vi "Experiment header-bundle basic image meta data.vi"(11 "AOL_Globals":T1 {"Plane Mode" items=["XY Plane", "XZ Plane", "YZ Plane", "arbitraryplane"]; "Frame Size" items=["100X100"=100, "128X128"=128, "200X200"=200, "256X256"=256, "512X512"=512, "1024x1024"=1024, "2048x2048"=2048]; "Back Apperture (mA)" format="%#.6g"; "Pockels (V)" format="%#.6g"; "PMT 2" format="%#.6g"; "PMT 1" format="%#.6g"; "Angle (degrees)" format="%#.6g"; "POI Dwell time (us)" format="%#.6g"}) -> (3 "Basic image meta-data":T7 {"Frame Size" items=["100X100"=100, "128X128"=128, "200X200"=200, "256X256"=256, "512X512"=512, "1024x1024"=1024, "2048x2048"=2048]})   [LabVIEW 2017]
uses:
  Typedefs/Header subclusters/Header params-Basic image meta data.ctl
  Typedefs/Frame Size.ctl
  Typedefs/Controls/AOL_Globals.ctl
  Typedefs/Imaging Protocols enum.ctl
  Typedefs/AOL modes.ctl
  Typedefs/Plane Mode.ctl
  Typedefs/Functional Mode.ctl
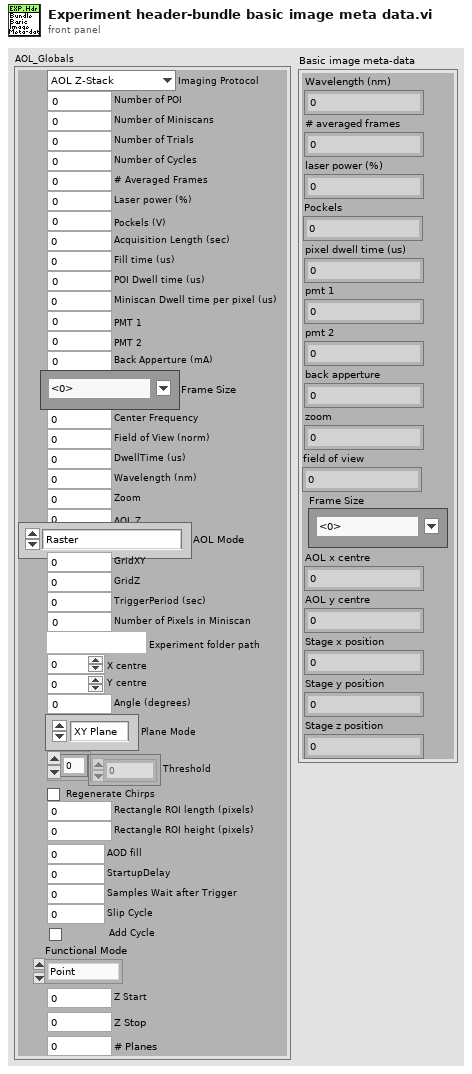
[diagram p1: front panel]
types:
  T1 = typedef "AOL_Globals.ctl" = cluster{"Imaging Protocol":T2, "Number of POI":u16, "Number of Miniscans":u16, "Number of Trials":u16, "Number of Cycles ":u64, "# Averaged Frames":u16, "Laser power (%)":u8, "Pockels (V)":dbl, "Acquisition Length (sec)":dbl, "Fill time (us)":dbl, "POI Dwell time (us)":dbl, "Miniscan Dwell time per pixel (us)":dbl, "PMT 1":dbl, "PMT 2":dbl, "Back Apperture (mA)":dbl, "Frame Size":T3, "Center Frequency":dbl, "Field of View (norm)":dbl, "DwellTime (us)":dbl, "Wavelength (nm)":dbl, "Zoom":dbl, "AOL Z":dbl, "AOL Mode":T4, "GridXY":dbl, "GridZ":dbl, "TriggerPeriod (sec)":dbl, "Number of Pixels in Miniscan":u16, "Experiment folder path":path, "X centre":dbl, "Y centre":dbl, "Angle (degrees)":dbl, "Plane Mode":T5, "Threshold":u16[], "Regenerate Chirps":bool, "Rectangle ROI length (pixels)":u16, "Rectangle ROI height (pixels)":u16, "AOD fill":u16, "StartupDelay":i32, "Samples Wait after Trigger":u16, "Slip Cycle":u32, "Add Cycle":bool, "Functional Mode":T6, "Z Start":dbl, "Z Stop":dbl, "# Planes":i32}
  T2 = typedef "Imaging Protocols enum.ctl" = enum16{"AOL Z-Stack", "Motor Z Stack", "Functional Acquisition", "Single Plane Acquisition", "Volume Acquisition", "Live Imaging", "Live Plane Imaging", "Live Volume Imaging"}
  T3 = typedef "Frame Size.ctl" = u16
  T4 = typedef "AOL modes.ctl" = enum16{"Raster", "Structural", "Pointing", "Mini Scan", "Alignment"}
  T5 = typedef "Plane Mode.ctl" = u16
  T6 = typedef "Functional Mode.ctl" = enum16{"Point", "Line", "Patch", "Plane", "Volume"}
  T7 = typedef "Header params-Basic image meta data.ctl" = cluster{"Wavelength (nm)":dbl, "# averaged frames":dbl, "laser power (%)":dbl, "Pockels":dbl, "pixel dwell time (us)":dbl, "pmt 1":dbl, "pmt 2":dbl, "back apperture":dbl, "zoom":dbl, "field of view":dbl, "Frame Size":T3, "AOL x centre":dbl, "AOL y centre":dbl, "Stage x position":dbl, "Stage y position":dbl, "Stage z position":dbl}
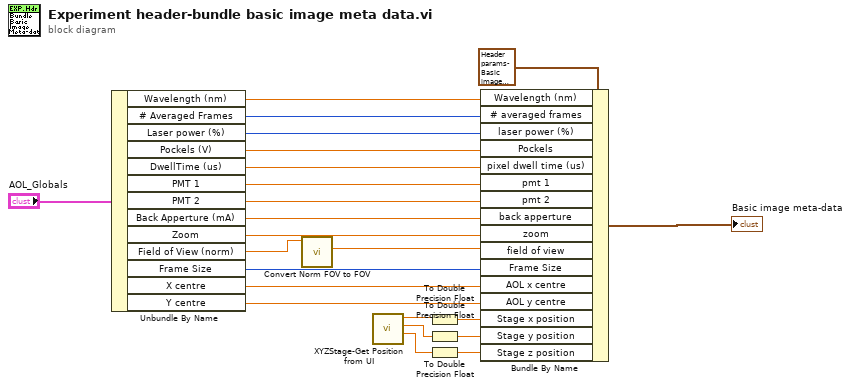
[diagram p0: block diagram]
diagram:
  n1 = Unbundle By Name("AOL_Globals") -> ("Wavelength (nm)"=w6:dbl, "# Averaged Frames"=w7:u16, "Laser power (%)"=w8:u8, "Pockels (V)"=w9:dbl, "DwellTime (us)"=w10:dbl, "PMT 1"=w11:dbl, "PMT 2"=w12:dbl, "Back Apperture (mA)"=w13:dbl, "Zoom"=w14:dbl, "Field of View (norm)"=w2:dbl, "Frame Size"=w3:T3, "X centre"=w15:dbl, "Y centre"=w16:dbl)
  n2 = call "Convert Norm FOV to FOV.vi"("Field of View(norm)"=w2) -> ("FOV"=w1:dbl)  [unwired: 9 in, 1 out]
  n3 = call "XYZStage-Get Position from UI.vi"() -> ("Z"=w22:sgl, "Y"=w21:sgl, "X"=w20:sgl)  [unwired: 8 in, 1 out]
  n4 = To Double Precision Float(number=w20) -> (double precision float=w17:dbl)
  n5 = To Double Precision Float(number=w21) -> (double precision float=w19:dbl)
  n6 = To Double Precision Float(number=w22) -> (double precision float=w18:dbl)
  n7 = Bundle By Name(cluster=T7 {"Wavelength (nm)"=0.0, "# averaged frames"=0.0, "laser power (%)"=0.0, "Pockels"=0.0, "pixel dwell time (us)"=0.0, "pmt 1"=0.0, "pmt 2"=0.0, "back apperture"=0.0, "zoom"=0.0, "field of view"=0.0, "Frame Size"=0, "AOL x centre"=0.0, "AOL y centre"=0.0, "Stage x position"=0.0, "Stage y position"=0.0, "Stage z position"=0.0} ("Basic image meta-data"), "Wavelength (nm)"=w6, "# averaged frames"=w7, "laser power (%)"=w8, "Pockels"=w9, "pixel dwell time (us)"=w10, "pmt 1"=w11, "pmt 2"=w12, "back apperture"=w13, "zoom"=w14, "field of view"=w1, "Frame Size"=w3, "AOL x centre"=w15, "AOL y centre"=w16, "Stage x position"=w17, "Stage y position"=w19, "Stage z position"=w18) -> (→"Basic image meta-data":T7)
